vi "Primary Buoyancy.vi"(6 "Primary Hot Density":dbl, 7 "Primary Cold Density":dbl, 9 "Primary Average Density":dbl, 10 "Pri Loop Height":dbl, 11 "MHX Length":dbl) -> (3 "Thermal Driving Pressure":dbl)   [LabVIEW 2019]
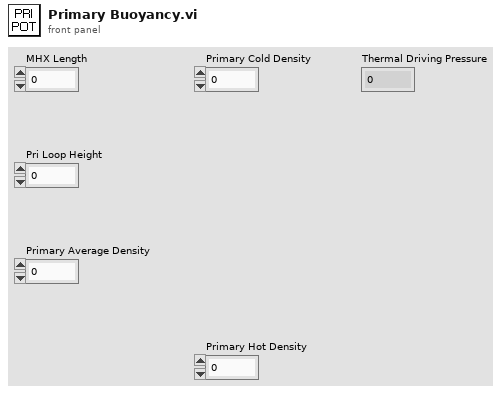
[diagram p1: front panel]
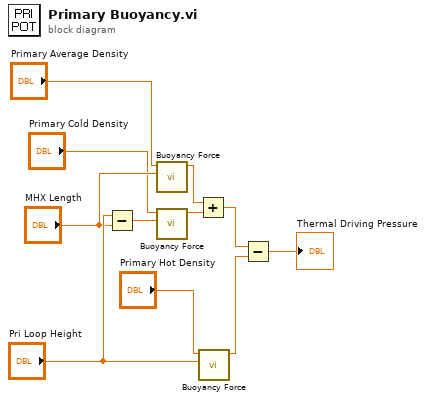
[diagram p0: block diagram]
diagram:
  n1 = Subtract(x="Pri Loop Height", y="MHX Length") -> (x-y=w4:dbl)
  n2 = call "Buoyancy Force.vi"("Height (m)"="MHX Length", "Density (kg/m^3)"="Primary Average Density") -> ("Potential (Pa)"=w6:dbl)  [unwired: 9 in]
  n3 = call "Buoyancy Force.vi"("Height (m)"=w4, "Density (kg/m^3)"="Primary Cold Density") -> ("Potential (Pa)"=w7:dbl)  [unwired: 9 in]
  n4 = Add(x=w6, y=w7) -> (x+y=w8:dbl)
  n5 = call "Buoyancy Force.vi"("Height (m)"="Pri Loop Height", "Density (kg/m^3)"="Primary Hot Density") -> ("Potential (Pa)"=w9:dbl)  [unwired: 9 in]
  n6 = Subtract(x=w8, y=w9) -> (x-y=→"Thermal Driving Pressure":dbl)
